vi "Stop Module.vi"(8 "error in":errorcluster, 9 "Wait for Module to stop? (F)":bool, 10 "Origin":string, 11 "Module ID":i32=-1) -> (0 "error out":errorcluster)   [LabVIEW 2023, in "Graph_data_collector.lvlib" / "Graph_UI.lvlib"]
doc: "Send the Stop request to the Module's Main.vi. If <b>Wait for Module to stop?</b> is TRUE, then this VI will not complete execution until the Module Main VI has stopped running.\n\n<b>Note:</b> If the cloneable module is running as singleton, then the 'Wait for Module to stop?' input is ignored... this VI will <b>always</b> wait until a cloneable Main VI running as singleton has stopped running.\n_____\nBased on DQMH Project Template 6.1.0.94."
uses:
  Graph_UI.lvlib
  Stop Argument--cluster.ctl
  Module Running State--enum.ctl
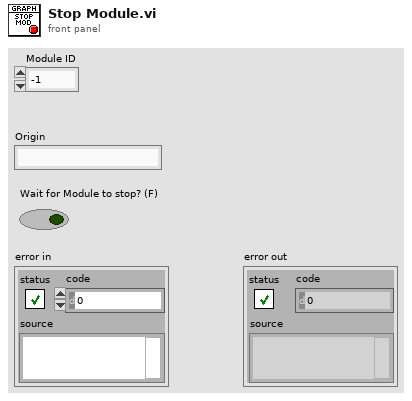
[diagram p1: front panel]
types:
  T1 = typedef "Graph_data_collector.lvlib/Graph_UI.lvlib/Module Running State--enum.ctl" = enum16{"Not Running", "Running as Cloneable", "Running as Singleton"}
  T2 = typedef "Graph_data_collector.lvlib/Graph_UI.lvlib/Stop Argument--cluster.ctl" = cluster{"Module ID":i32, "Origin":string, "Exit via Stop Module Req?":bool, "Wait for Module to stop?":bool}
  T3 = typedef "Graph_data_collector.lvlib/Graph_UI.lvlib/Request Events--cluster.ctl" = cluster{"Stop Module":refnum<user-event>, "Show Panel":refnum<user-event>, "Hide Panel":refnum<user-event>, "Show Diagram":refnum<user-event>, "Get Module Execution Status":refnum<user-event>, "New Data":refnum<user-event>, "SetP":refnum<user-event>}
  T4 = enum32{"Bad", "Idle", "Run top level", "Running"}
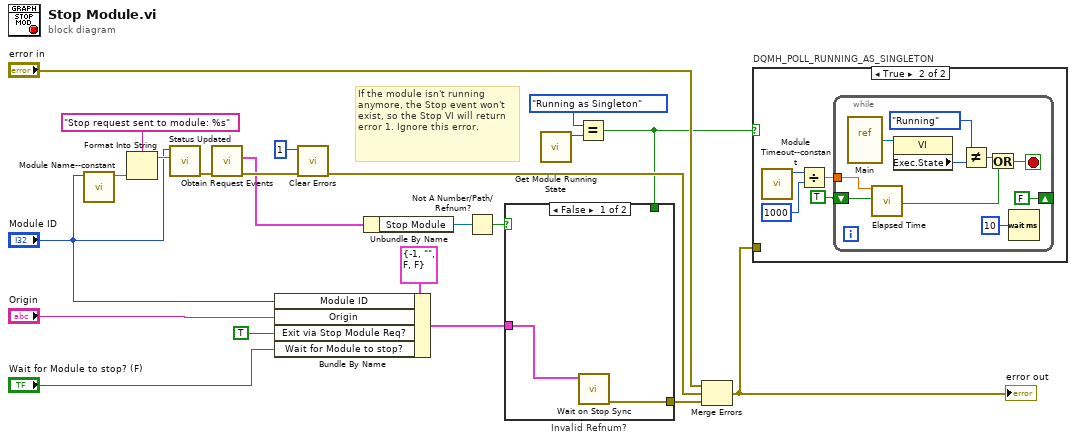
[diagram p0: block diagram]
diagram:
  # "If the module isn't running anymore, the Stop event won't exist, so the Stop VI will return error 1. Ignore this error."
  n1 = call "Module Name--constant.vi"("Module ID"="Module ID") -> ("Module Name"=w19:string)  [unwired: 10 in]
  n2 = Format Into String(format string="Stop request sent to module: %s", w19) -> (resulting string=w20:string)  [unwired: 2 in, 1 out]
  n3 = call "Status Updated.vi"("Status"=w20, "Module ID"="Module ID") -> ("error out"=w13:errorcluster)  [unwired: 9 in]
  n4 = call "Obtain Request Events.vi"("error in (no error)"=w13) -> ("error out"=w12:errorcluster, "Graph_UI Request Events"=w10:T3)  [unwired: 9 in]
  n5 = Bundle By Name(cluster=T2 {"Module ID"=-1, "Origin"="", "Exit via Stop Module Req?"=FALSE, "Wait for Module to stop?"=FALSE} ("event data"), "Module ID"="Module ID", "Origin"="Origin", "Exit via Stop Module Req?"=TRUE, "Wait for Module to stop?"="Wait for Module to stop? (F)") -> (w14:T2)
  n6 = call <vilib>:"Clear Errors.vi"("error in (no error)"=w12, "specific error code to clear (0: all)"=1) -> ("error out"=w9:errorcluster)  [unwired: 4 in, 1 out]
  n7 = Unbundle By Name(w10) -> ("Stop Module"=w15:refnum<user-event>)
  n8 = Not A Number/Path/Refnum?(number/path/refnum=w15) -> (NaN/Path/Refnum?=w16:bool)
  n9 = call "Get Module Running State.vi"() -> ("Module Running State"=w5:T1)  [unwired: 11 in]
  n10 = Equal?(x=Module_Running_State--enum."Running as Singleton", y=w5) -> (x = y?=w4:bool)
  n11 = case "Invalid Refnum?" shown="False" w16 {
    tunnel: [w24 _] -> w8
    tunnel: w14 -> [w23 _]
    tunnel: w4 -> [_ _]
    frame False {
      n12 = call "Wait on Stop Sync.vi"("Stop Argument"=w23) -> ("error out"=w24:errorcluster)  [unwired: 10 in]
    }
    frame True {
      # "Module is exiting. No need to send the standard \"not running\" error that is sent in other request VIs."
    }
  }
  n13 = Merge Errors("error in", w9, w8) -> (w2:errorcluster)
  "error out" <- w2
  n14 = case "DQMH_POLL_RUNNING_AS_SINGLETON" shown="True" w4 {
    tunnel: w2 -> [_ _]
    frame False {
    }
    frame True {
      n15 = call "Module Timeout--constant.vi"() -> ("Module Timeout"=w28:i32)  [unwired: 11 in]
      n16 = Divide(x=w28, y=1000) -> (x/y=w26:dbl)
      n17 = while {
        tunnel: w26 -> [w31]
        shift-right: [FALSE] -> _
        shift-left: TRUE -> [w32]
        stop <- w34 stop-if-true
        n18 = vi-ref "Main.vi"() -> (w38:refnum<vi>)
        n19 = call "Elapsed Time"("Time Target (s)"=w31, "Reset"=w32) -> ("Time has Elapsed"=w30:bool)  [unwired: 10 in, 7 out]
        n20 = property class="VI"(reference=w38) -> ("Exec.State"=w37:T4)  [unwired: 1 in, 2 out]
        n21 = Not Equal?(x=T4."Running", y=w37) -> (x != y?=w35:bool)
        n22 = Or(x=w35, y=w30) -> (x .or. y?=w34:bool)
        n23 = Wait (ms)(milliseconds to wait=u32 10) -> ()  [unwired: 1 out]
      }
    }
  }
